vi "Read Key.vi"(8 "Error In":errorcluster, 11 "Section In":refnum<class "Section.lvclass">) -> (0 "Error Out":errorcluster, 2 "Key":string, 3 "Section Out":refnum<class "Section.lvclass">)   [LabVIEW 2018, in "Toolkit.lvlib" / "Nodes.lvlib" / "Section.lvclass"]
uses:
  Section.lvclass
  Section.lvclass/Section.ctl
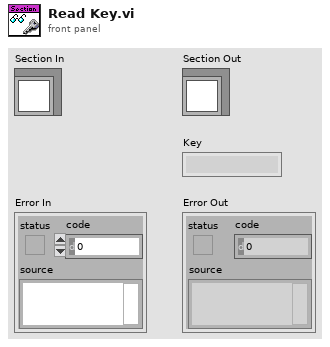
[diagram p1: front panel]
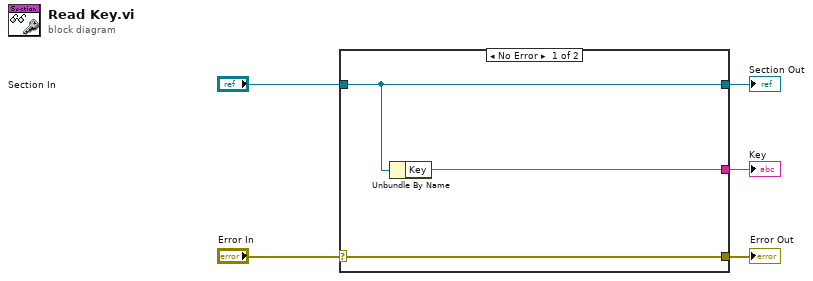
[diagram p0: block diagram]
diagram:
  n1 = case shown="No Error" "Error In" {
    selector: "Error In" -> [w8 w9]
    tunnel: [w8 w9] -> w4
    tunnel: [w7 w10] -> w2
    tunnel: "Section In" -> [w7 w10]
    tunnel: [w6 _] -> w1
    frame No Error {
      n2 = Unbundle By Name(w7) -> ("Key"=w6:string)
    }
    frame Error {
    }
  }
  "Error Out" <- w4
  "Section Out" <- w2
  "Key" <- w1
